vi "Read measure (Multi-Channel F, P1 and P2).vi"(8 "error in":errorcluster, 11 "MB_TCP session in":refnum<class "MB_Master_TCP.lvclass">) -> (0 "error out":errorcluster, 1 "Fmeasure (F, P1, P2)":T1, 3 "MB session out":refnum<class "MB_Master_TCP.lvclass">)   [LabVIEW 2024, in "Bronkhorst Flexi-Flow ModbusTCP API.lvlib"]
uses:
  Bronkhorst Flexi-Flow ModbusTCP API.lvlib
  <vilib>/Plasmionique/MB Master/MB_Master_TCP/MB_Master_TCP.lvclass
  Fmeasure (F,P1,P2)--cluster.ctl
  PDU Address Float 32-bit Params--ring.ctl
  Read Float Register.vi
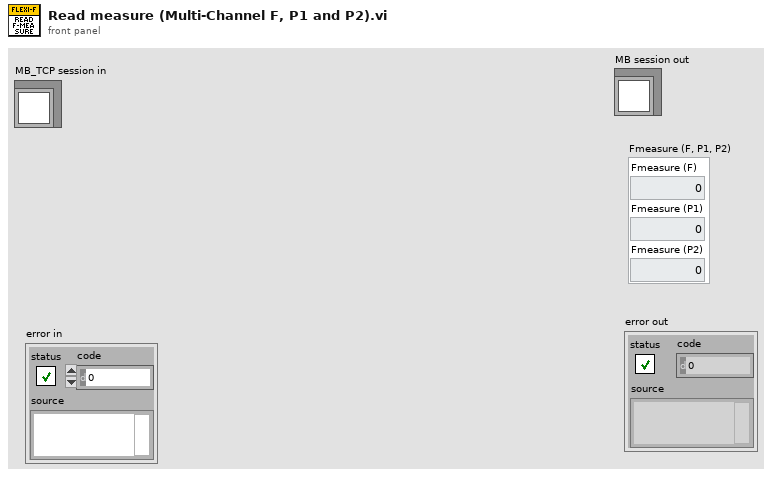
[diagram p1: front panel]
types:
  T1 = typedef "Bronkhorst Flexi-Flow ModbusTCP API.lvlib/Fmeasure (F,P1,P2)--cluster.ctl" = cluster{"Fmeasure (F)":sgl, "Fmeasure (P1)":sgl, "Fmeasure (P2)":sgl}
  T2 = typedef "Bronkhorst Flexi-Flow ModbusTCP API.lvlib/PDU Address Float 32-bit Params--ring.ctl" = u16
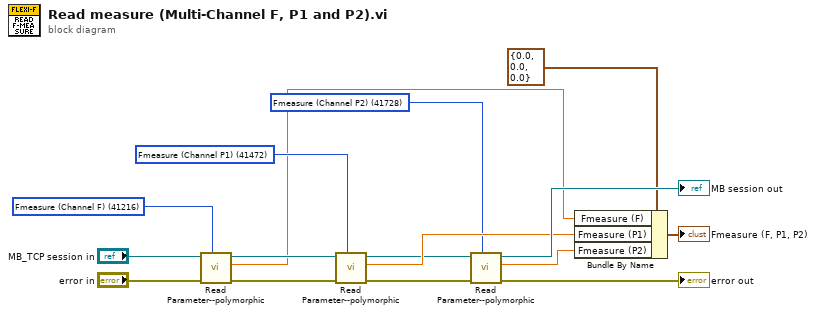
[diagram p0: block diagram]
diagram:
  w12 = T2 41472 items=["FSetpoint (Channel F)"=41240, "Fmeasure (Channel F)"=41216, "FSetpoint (Channel P1)"=41496, "Fmeasure (Channel P1)"=41472, "FSetpoint (Channel P2)"=41752, "Fmeasure (Channel P2)"=41728, "Capacity 0%"=41392, "Counter limit (Float)"=59416, "Inlet Pressure"=61801, "Outlet Pressure"=61809, "PID-Kp"=62120, "PID-Ti"=62128, "PID-Td"=62136, "Dynamic display factor"=62728, "Static display factor"=62736, "Exponential smoothing"=62752] ("PDU Address 32-bit Float")
  w1 = T2 41728 items=["FSetpoint (Channel F)"=41240, "Fmeasure (Channel F)"=41216, "FSetpoint (Channel P1)"=41496, "Fmeasure (Channel P1)"=41472, "FSetpoint (Channel P2)"=41752, "Fmeasure (Channel P2)"=41728, "Capacity 0%"=41392, "Counter limit (Float)"=59416, "Inlet Pressure"=61801, "Outlet Pressure"=61809, "PID-Kp"=62120, "PID-Ti"=62128, "PID-Td"=62136, "Dynamic display factor"=62728, "Static display factor"=62736, "Exponential smoothing"=62752] ("PDU Address 32-bit Float")
  w16 = T2 41216 items=["FSetpoint (Channel F)"=41240, "Fmeasure (Channel F)"=41216, "FSetpoint (Channel P1)"=41272, "Fmeasure (Channel P1)"=41248, "FSetpoint (Channel P2)"=41304, "Fmeasure (Channel P2)"=41280, "Capacity 0%"=41392, "Counter limit (Float)"=59416, "Inlet Pressure"=61801, "Outlet Pressure"=61809, "PID-Kp"=62120, "PID-Ti"=62128, "PID-Td"=62136, "Dynamic display factor"=62728, "Static display factor"=62736, "Exponential smoothing"=62752] ("PDU Address 32-bit Float")
  n1 = call-poly "Read Parameter--polymorphic.vi"("PDU Address 32-bit Float"=w16, "error in"="error in", "MB_TCP session in"="MB_TCP session in") -> ("error out"=w13:errorcluster, "Value"=w6:sgl, "MB session out"=w11:refnum<class "MB_Master_TCP.lvclass">)  [unwired: 6 in]
  n2 = call-poly "Read Parameter--polymorphic.vi"("PDU Address 32-bit Float"=w12, "error in"=w13, "MB_TCP session in"=w11) -> ("error out"=w9:errorcluster, "Value"=w5:sgl, "MB session out"=w3:refnum<class "MB_Master_TCP.lvclass">)  [unwired: 6 in]
  n3 = call-poly "Read Parameter--polymorphic.vi"("PDU Address 32-bit Float"=w1, "error in"=w9, "MB_TCP session in"=w3) -> ("error out"=→"error out":errorcluster, "Value"=w4:sgl, "MB session out"=→"MB session out":refnum<class "MB_Master_TCP.lvclass">)  [unwired: 6 in]
  n4 = Bundle By Name(cluster=T1 {"Fmeasure (F)"=0.0, "Fmeasure (P1)"=0.0, "Fmeasure (P2)"=0.0}, "Fmeasure (F)"=w6, "Fmeasure (P1)"=w5, "Fmeasure (P2)"=w4) -> (→"Fmeasure (F, P1, P2)":T1)
